vi "change tag raw default value.vi"(7 "owner ID":string, 8 "error in":errorcluster, 9 "raw default":string, 10 "tag name":string, 11 "engine configuration in":refnum<class "engine configuration.lvclass">) -> (0 "error out":errorcluster, 3 "engine configuration out":refnum<class "engine configuration.lvclass">)   [LabVIEW 2014, in "engine configuration.lvclass"]
doc: "This function updates the raw default value of a tag."
uses:
  engine configuration.lvclass
  <vilib>/NI/Tag Bus/tag/tag descriptor.lvclass
  <vilib>/NI/Tag Bus/tag/tag descriptor.lvclass/tag descriptor.ctl
  engine configuration.lvclass/engine configuration.ctl
  <vilib>/NI/Tag Bus/tag/write tag name.vi
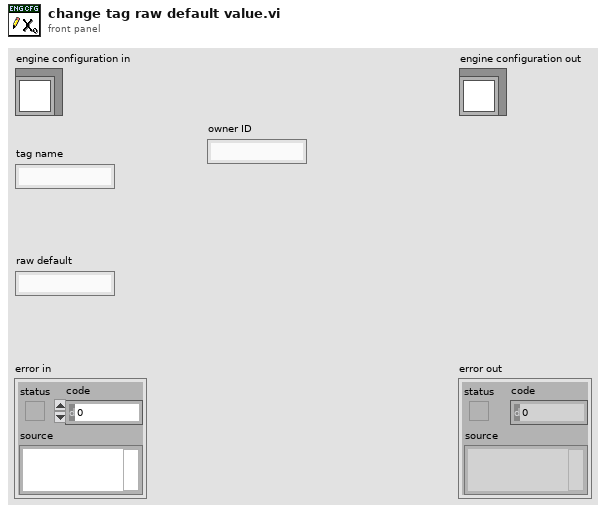
[diagram p1: front panel]
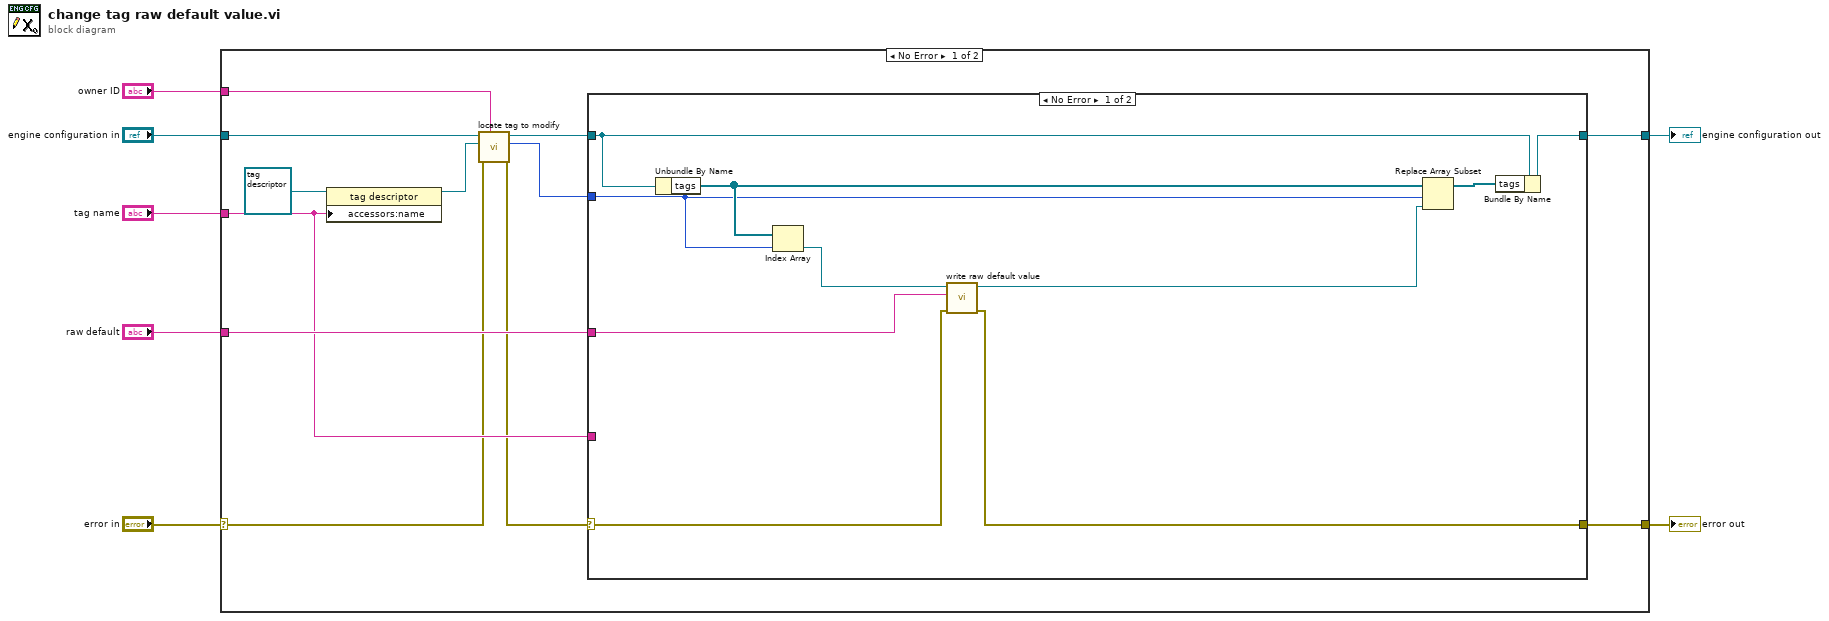
[diagram p0: block diagram]
diagram:
  n1 = case shown="No Error" "error in" {
    selector: "error in" -> [w10 w33]
    tunnel: [w17 w33] -> w6
    tunnel: [w18 w32] -> w4
    tunnel: "engine configuration in" -> [w14 w32]
    tunnel: "tag name" -> [w15 _]
    tunnel: "raw default" -> [w16 _]
    tunnel: "owner ID" -> [w11 _]
    frame No Error {
      n2 = property class="tag descriptor"(reference=refnum<class "tag descriptor.lvclass"> refnum ("tag descriptor"), "accessors:name"=w15) -> (reference out=w12:refnum<class "tag descriptor.lvclass">)  [unwired: 1 in, 1 out]
      n3 = call "locate tag to modify.vi"("owner ID"=w11, "error in"=w10, "tag descriptor"=w12, "engine configuration in"=w14) -> ("error out"=w9:errorcluster, "index"=w8:i32, "engine configuration out"=w13:refnum<class "engine configuration.lvclass">)  [unwired: 5 in]
      n4 = case shown="No Error" w9 {
        selector: w9 -> [w21 w30]
        tunnel: w13 -> [w26 w31]
        tunnel: [w27 w31] -> w18
        tunnel: [w20 w30] -> w17
        tunnel: w16 -> [w24 _]
        tunnel: w15 -> [_ _]
        tunnel: w8 -> [w25 _]
        frame No Error {
          n5 = Unbundle By Name(w26) -> ("tags"=w29:refnum<class "tag descriptor.lvclass">[])
          n6 = Index Array(array=w29, index=w25) -> (element=w22:refnum<class "tag descriptor.lvclass">)
          n7 = call <vilib>:"write raw default value.vi"("error in"=w21, "raw default"=w24, "system tag in"=w22) -> ("error out"=w20:errorcluster, "system tag out"=w23:refnum<class "tag descriptor.lvclass">)  [unwired: 7 in]
          n8 = Replace Array Subset(array=w29, new element=w23, index=w25) -> (w28:refnum<class "tag descriptor.lvclass">[])
          n9 = Bundle By Name(cluster=w26, "tags"=w28) -> (w27:refnum<class "engine configuration.lvclass">)
        }
        frame Error {
        }
      }
    }
    frame Error {
    }
  }
  "error out" <- w6
  "engine configuration out" <- w4
